vi "Read Data Raw.vi"(8 "error in (no error)":errorcluster, 11 "Experiment in":refnum<class "Experiment.lvclass">) -> (0 "error out":errorcluster, 2 "Data Raw":i32[][][][](array[numeric]), 3 "Experiment out":refnum<class "Experiment.lvclass">)   [LabVIEW 2019, in "Experiment.lvclass"]
uses:
  Experiment.lvclass
  Experiment.lvclass/Experiment.ctl
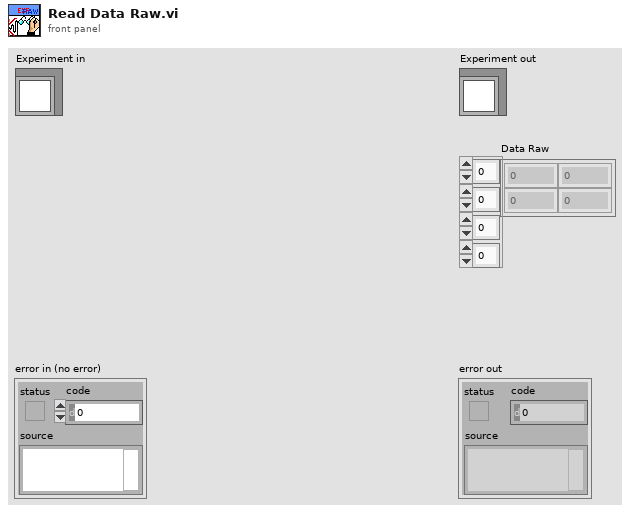
[diagram p1: front panel]
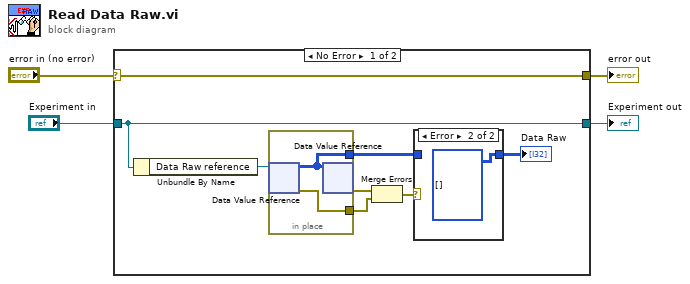
[diagram p0: block diagram]
diagram:
  n1 = case shown="No Error" "error in (no error)" {
    selector: "error in (no error)" -> [w12 w17]
    tunnel: [w12 w17] -> w3
    tunnel: [w11 w18] -> w1
    tunnel: "Experiment in" -> [w11 w18]
    frame No Error {
      n2 = Unbundle By Name(w11) -> ("Data Raw reference"=w10:refnum<data-value>)
      n3 = in-place {
        in-place-border: [w16] -> w8
        in-place-border: [w15] -> w6
        n4 = in-place-dvr #1(w10) -> (w15:i32[][][][], w16:errorcluster)
        n5 = in-place-dvr #1(w15) -> (w9:errorcluster)  [unwired: 1 out]
      }
      n6 = Merge Errors(w9, w8) -> (w7:errorcluster)
      n7 = case shown="Error" w7 {
        tunnel: w6 -> [w13 _]
        tunnel: [w13 i32[][][][] [] ("Data raw")] -> w5
        frame No Error {
        }
        frame Error {
        }
      }
      "Data Raw" <- w5
    }
    frame Error {
    }
  }
  "error out" <- w3
  "Experiment out" <- w1
